vi "Control_Panel_Execute.vi"() -> ()   [LabVIEW 2019]
uses:
  Control_Panel_Globals.vi
  Globals/Solenoid Globals.vi
  <vilib>/Rock Robotics/WPI/ThirdParty/REV Robotics/SPARK MAX/Typedef/Spark MAX Control Type.ctl
  <vilib>/Rock Robotics/WPI/Solenoid/WPI_SolenoidValue.ctl
  <vilib>/Rock Robotics/WPI/Solenoid/WPI_SolenoidSetEnum.vi
  Control_Panel_States.ctl
  Control_Panel_Cluster.ctl
panel:
  in  "time_to_run":u32
  in  "Spinwheel_Throttle":dbl
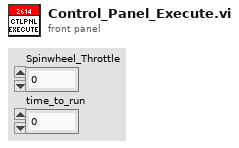
[diagram p1: front panel]
types:
  T1 = typedef "WPI_MotorControlDeviceRef.ctl" = cluster{"DeviceStatus":errorcluster, "Type":T2, "PWM":cluster{"PWM Channel":T3, "DeadBand":T4}, "CAN":cluster{"Device Number":u8, "SetOutput VI Ref":variant, "GetOutput VI Ref":variant, "Enable VI Ref":variant, "Disable VI Ref":variant, "Data":variant}, "Invert":bool, "DIO PWM":cluster{"PWM \"Enable\" Channel":T3, "DIOChannel":T5, "PWM Rate":dbl}}
  T2 = typedef "WPI_MotorControlType.ctl" = enum16{"PWM", "CAN", "DIO PWM"}
  T3 = typedef "FPGA_DIOPWMChannel.ctl" = enum8{"PWM 0", "PWM 1", "PWM 2", "PWM 3", "PWM 4", "PWM 5", "PWM 6", "PWM 7", "PWM 8", "PWM 9", "PWM MXP 0", "PWM MXP 1", "PWM MXP 2", "PWM MXP 3", "PWM MXP 4", "PWM MXP 5", "PWM MXP 6", "PWM MXP 7", "PWM MXP 8", "PWM MXP 9", "Invalid"}
  T4 = typedef "WPI_PWMDeadband.ctl" = cluster{"Name":string, "maxPositivePwm":i32, "minPositivePwm":i32, "centerPwm":i32, "maxNegativePwm":i32, "minNegativePwm":i32, "angularRange":u16}
  T5 = typedef "FPGA_DIOChannel.ctl" = enum8{"DIO 0", "DIO 1", "DIO 2", "DIO 3", "DIO 4", "DIO 5", "DIO 6", "DIO 7", "DIO 8", "DIO 9", "DIO MXP 0", "DIO MXP 1", "DIO MXP 2", "DIO MXP 3", "DIO MXP 4", "DIO MXP 5", "DIO MXP 6", "DIO MXP 7", "DIO MXP 8", "DIO MXP 9", "DIO MXP 10", "DIO MXP 11", "DIO MXP 12", "DIO MXP 13", "DIO MXP 14", "DIO MXP 15", "SPI Port CS1", "SPI Port CS2", "SPI Port CS3", "SPI Port MISO", "SPI Port MOSI", "Invalid"}
  T6 = typedef "WPI_SolenoidDevRef.ctl" = cluster{"DevStatus":errorcluster, "Pneumatics Control Module":u8, "Forward Solenoid Channel":T7, "Reverse Solenoid Channel":T7}
  T7 = typedef "WPI_SolenoidChannel.ctl" = enum8{"Solenoid 0", "Solenoid 1", "Solenoid 2", "Solenoid 3", "Solenoid 4", "Solenoid 5", "Solenoid 6", "Solenoid 7", "Invalid"}
  T8 = typedef "WPI_SolenoidValue.ctl" = enum16{"Off", "On", "Forward", "Reverse"}
  T9 = typedef "Control_Panel_Cluster.ctl" = cluster{"Control_State":T10, "Start_Movement":bool, "Abort":bool, "Rotation_Control?":bool, "Positional_Control? ":bool, "Throttle":dbl, "Extend?":bool}
  T10 = typedef "Control_Panel_States.ctl" = enum16{"No-Op", "Rotational_Control", "Positional_Control", "Manual_Control"}
  T11 = typedef "Spark MAX Control Type.ctl" = enum16{"Percent VBus", "Voltage", "Velocity", "Position", "Smart Motion", "Current", "Smart Velocity"}
  T12 = typedef "Control_Panel_Cluster.ctl" = cluster{"Control_State":T10, "Start_Movement":bool, "Abort":bool, "Rotation_Control?":bool, "Positional_Control? ":bool, "Throttle":dbl}
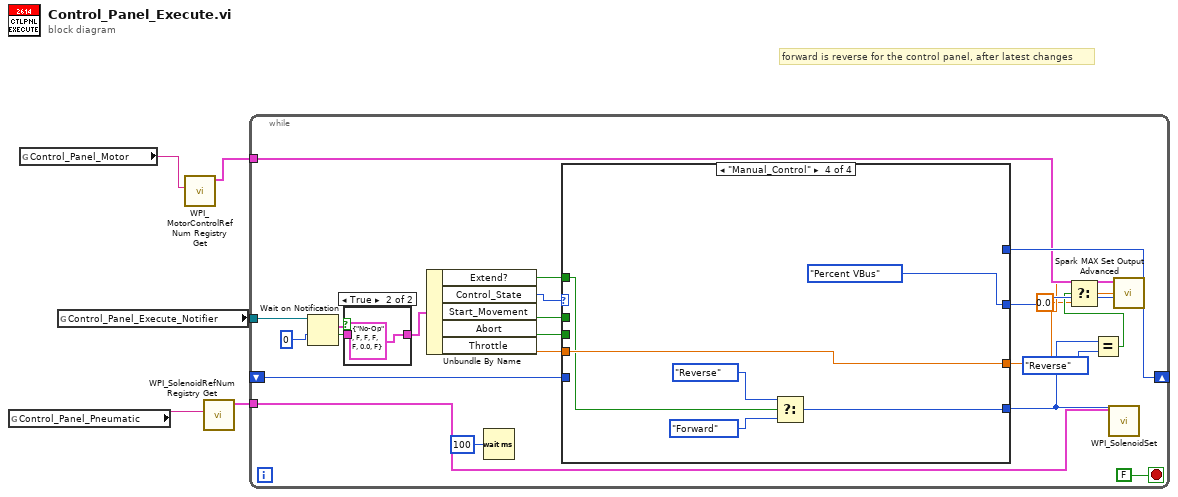
[diagram p0: block diagram]
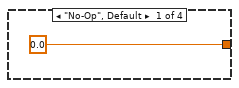
[diagram p3: hidden frame]
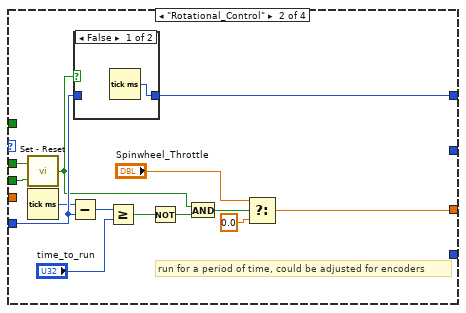
[diagram p4: hidden frame]
diagram:
  # "forward is reverse for the control panel, after latest changes"
  n1 = global read "Solenoid Globals.vi" "Control_Panel_Pneumatic"() -> (w4:string)
  n2 = global read "Control_Panel_Globals.vi" "Control_Panel_Motor"() -> (w2:string)
  n3 = global read "Control_Panel_Globals.vi" "Control_Panel_Execute_Notifier"() -> (w5:refnum<notifier>)
  n4 = call <vilib>:"WPI_MotorControlRefNum Registry Get.vi"("refnum name"=w2) -> ("MotorControlDevRef"=w1:T1)  [unwired: 9 in, 1 out]
  n5 = call <vilib>:"WPI_SolenoidRefNum Registry Get.vi"("refnum name"=w4) -> ("SolenoidDevRef"=w3:T6)  [unwired: 9 in, 1 out]
  n6 = while {
    tunnel: w5 -> [w28]
    shift-right: [w24] -> _
    shift-left: _ -> [w23]
    tunnel: w3 -> [w20]
    tunnel: w1 -> [w19]
    stop <- FALSE stop-if-true
    n7 = Wait on Notification(notifier=w28, timeout in ms (-1)=0) -> (notification=w7:T12, timed out?=w8:bool)  [unwired: 2 in, 2 out]
    n8 = case shown="True" w8 {
      tunnel: w7 -> [w29 _]
      tunnel: [w29 T9 {"Control_State"=enum."No-Op", "Start_Movement"=FALSE, "Abort"=FALSE, "Rotation_Control?"=FALSE, "Positional_Control? "=FALSE, "Throttle"=0.0, "Extend?"=FALSE} ("Control_Panel_Cluster")] -> w6
      frame False {
      }
      frame True {
      }
    }
    n9 = Unbundle By Name(w6) -> ("Extend?"=w10:bool, "Control_State"=w17:T10, "Start_Movement"=w26:bool, "Abort"=w25:bool, "Throttle"=w27:dbl)
    n10 = Wait (ms)(milliseconds to wait=u32 100) -> ()  [unwired: 1 out]
    n11 = case shown="\"Manual_Control\"" w17 {
      tunnel: [0.0 ("Spin_Wheel_Speed") w32 _ w53] -> w13
      tunnel: w27 -> [_ _ _ w53]
      tunnel: w26 -> [_ w45 _ _]
      tunnel: w25 -> [_ w44 _ _]
      tunnel: [_ w42 _ _] -> w24
      tunnel: w23 -> [_ w39 _ _]
      tunnel: [_ _ _ Spark_MAX_Control_Type."Percent VBus" ("Control Mode")] -> w18
      tunnel: [_ _ _ w51] -> w11
      tunnel: w10 -> [_ _ _ w50]
      frame "No-Op", Default {
      }
      frame "Rotational_Control" {
        # "run for a period of time, could be adjusted for encoders"
        n12 = call "Set - Reset.vi"("Reset"=w44, "Set"=w45) -> ("Output"=w37:bool)
        n13 = Tick Count (ms)() -> (millisecond timer value=w38:u32)
        n14 = Subtract(x=w38, y=w39) -> (x-y=w41:u32)
        n15 = case shown="False" w37 {
          tunnel: [w46 w47] -> w42
          tunnel: w39 -> [_ w47]
          frame False {
            n16 = Tick Count (ms)() -> (millisecond timer value=w46:u32)
          }
          frame True {
          }
        }
        n17 = Greater Or Equal?(x=w41, y="time_to_run") -> (x >= y?=w36:bool)
        n18 = Not(x=w36) -> (.not. x?=w35:bool)
        n19 = And(x=w37, y=w35) -> (x .and. y?=w34:bool)
        n20 = Select(t="Spinwheel_Throttle", s=w34, f=0.0) -> (s? t:f=w32:dbl)
      }
      frame "Positional_Control" {
        # "SPINNING LOGIC, color offsets"
      }
      frame "Manual_Control" {
        n21 = Select(t=WPI_SolenoidValue."Reverse" ("y"), s=w50, f=WPI_SolenoidValue."Forward" ("y")) -> (s? t:f=w51:T8)
      }
    }
    n22 = Equal?(x=w11, y=WPI_SolenoidValue."Reverse") -> (x = y?=w14:bool)
    n23 = Select(t=w13, s=w14, f=0.0) -> (s? t:f=w15:dbl)
    n24 = call-poly <vilib>:"WPI_SolenoidSet.vi"("Value"=w11, "SolenoidDevRef"=w20) -> ()  [unwired: 8 in, 2 out]
    n25 = call <vilib>:"Spark MAX Set Output Advanced.vi"("Control Mode"=w18, "Setpoint"=w15, "MotorControlDevRef"=w19) -> ()  [unwired: 7 in, 2 out]
  }
